vi "CalculAngle.vi"(8 "error constant":errorcluster, 9 "Zaxis":dbl, 10 "Yaxis":dbl, 11 "Xaxis":dbl) -> (0 "error constant 2":errorcluster, 3 "Numeric":dbl)   [LabVIEW 2019]
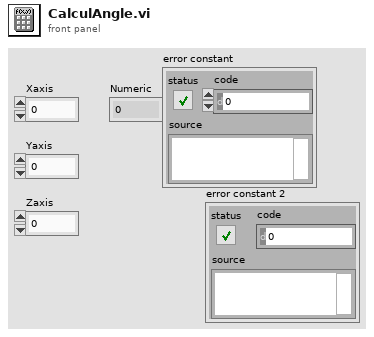
[diagram p1: front panel]
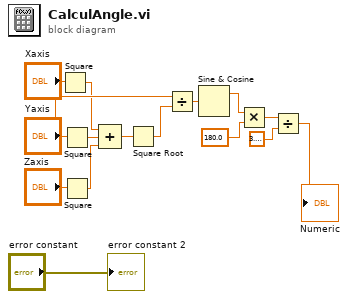
[diagram p0: block diagram]
diagram:
  n1 = Square(x="Xaxis") -> (x^2=w3:dbl)
  n2 = Square(x="Yaxis") -> (x^2=w4:dbl)
  n3 = Square(x="Zaxis") -> (x^2=w5:dbl)
  n4 = Compound Arithmetic op=ADD(w3, w4, w5) -> (w2:dbl)
  n5 = Square Root(x=w2) -> (sqrt(x)=w8:dbl)
  n6 = Divide(x="Yaxis", y=w8) -> (x/y=w10:dbl)
  n7 = Sine & Cosine(0:w10) -> (1:w11:dbl)  [unwired: 1 out]
  n8 = Multiply(x=w11, y=180.0) -> (x*y=w13:dbl)
  n9 = Divide(x=w13, y=3.141592653589793) -> (x/y=→"Numeric":dbl)
  "error constant 2" <- "error constant"
